vi "Shutdown.vi"(8 "error in (no error)":errorcluster, 11 "CD_Process in":refnum<class "CD_Process.lvclass">) -> (0 "error out":errorcluster, 3 "CD_Process out":refnum<class "CD_Process.lvclass">)   [LabVIEW 2019, in "TimingDRV Engine.lvlib" / "CD_Process.lvclass"]
uses:
  CD_Process.lvclass
  CD_Process.lvclass/CD_Process.ctl
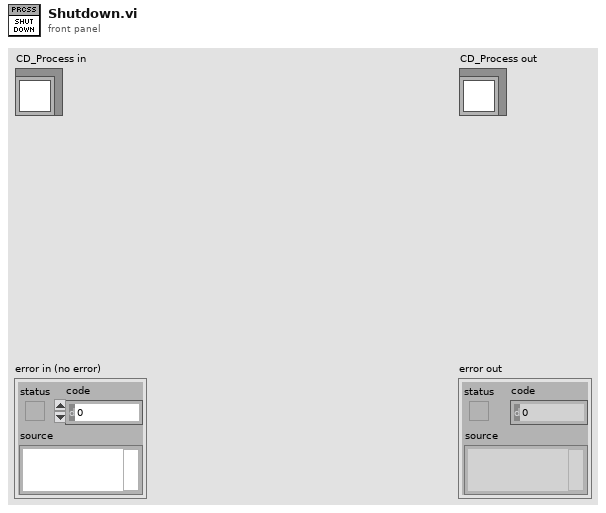
[diagram p1: front panel]
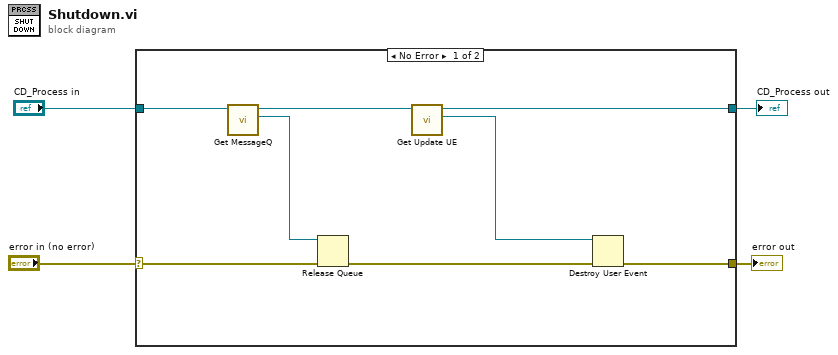
[diagram p0: block diagram]
diagram:
  n1 = case shown="No Error" "error in (no error)" {
    selector: "error in (no error)" -> [w11 w14]
    tunnel: [w5 w14] -> w3
    tunnel: [w6 w13] -> w1
    tunnel: "CD_Process in" -> [w12 w13]
    frame No Error {
      n2 = call "Get MessageQ.vi"("CD_Process in"=w12) -> ("MessageQ"=w10:refnum<queue>, "CD_Process out"=w9:refnum<class "CD_Process.lvclass">)  [unwired: 9 in]
      n3 = Release Queue(queue=w10, error in (no error)=w11) -> (error out=w8:errorcluster)  [unwired: 1 in, 2 out]
      n4 = call "Get Update UE.vi"("CD_Process in"=w9) -> ("Update UE"=w7:refnum<user-event>, "CD_Process out"=w6:refnum<class "CD_Process.lvclass">)  [unwired: 9 in]
      n5 = Destroy User Event(user event=w7, error in=w8) -> (error out=w5:errorcluster)
    }
    frame Error {
    }
  }
  "error out" <- w3
  "CD_Process out" <- w1
